vi "Controller test.vi"() -> ()   [LabVIEW 2018]
doc: "Test-bench for the various controllers and discrete transfer functions."
uses:
  TypeDefs/Select_TF.ctl
  <vilib>/Platform/TimedLoop/XDataNode/timing_clust.ctl
  <vilib>/Platform/TimedLoop/XDataNode/nitl_modes.ctl
  <vilib>/Platform/TimedLoop/XDataNode/wakeup.ctl
  Controllers/TF_diff_mode.ctl
  <vilib>/platform/TimedLoop/XDataNode/XDataNode.xnode
  <vilib>/Platform/TimedLoop/XDataNode/XDNodeRunTimeDep.lvlib
  Controllers/DiscreteControllers.lvlib
  <vilib>/ptbypt/NI_PtbyPt.lvlib
panel:
  in  "Select discrete \ntransfer function":T1
  out "#Loops late":i16
  in  "stop":bool
  out "System Waveform Chart":cluster{"square wave":dbl, "Output":dbl}(graph)
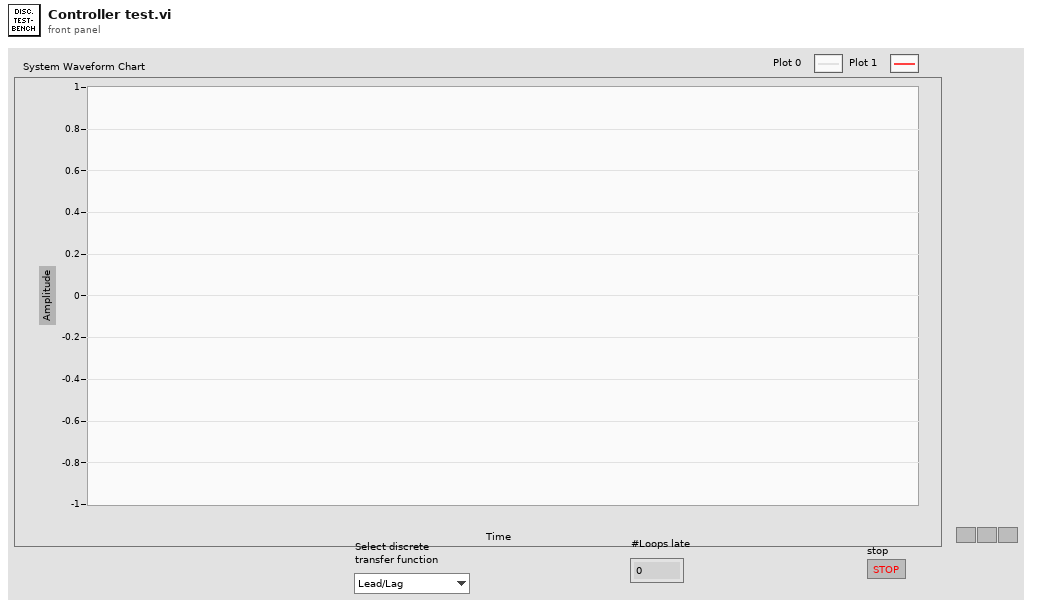
[diagram p1: front panel]
types:
  T1 = typedef "Select_TF.ctl" = enum16{"Lead/Lag", "Gain=20", "Unity", "Integrator"}
  T2 = typedef "XDNodeRunTimeDep.lvlib/timing_clust.ctl" = cluster{"Expected End [f-1]":u64, "Actual End [f-1]":u64, "Finished Late? [f-1]":bool, "Expected End [i-1]":u64, "Actual End [i-1]":u64, "Finished Late? [i-1]":bool, "Expected Start [i]":u64, "Actual Start [i]":u64, "Expected Start [f]":u64, "Actual Start [f]":u64, "Source Name":string, "Structure Name":string, "Period":i64, "Deadline":i64, "Offset":i64, "Start":i64, "Priority":i32, "Timeout":i32, "Mode":T3, "Wakeup Reason":T4, "Error":errorcluster, "Source Type":string, "Secondary Source Type":string, "Global End Time":u64, "Global Start Time":u64, "Frame Duration":u64, "Iteration Duration":u64, "Assigned CPU":i32, "I/O Scan Engine Mode":u32}
  T3 = typedef "XDNodeRunTimeDep.lvlib/nitl_modes.ctl" = enum32{"No Change", "Process missed periods, maintain original phase", "Discard missed periods, maintain original phase", "Process missed periods, ignore original phase", "Discard missed periods, ignore original phase"}
  T4 = typedef "XDNodeRunTimeDep.lvlib/wakeup.ctl" = enum32{"Normal", "Aborted", "Asynchronous wakeup", "Timing source error", "Timed loop error", "Timeout"}
  T5 = typedef "DiscreteControllers.lvlib/TF_diff_mode.ctl" = enum16{"Forward Euler", "Backward Euler", "Tustin (Bilinear)"}
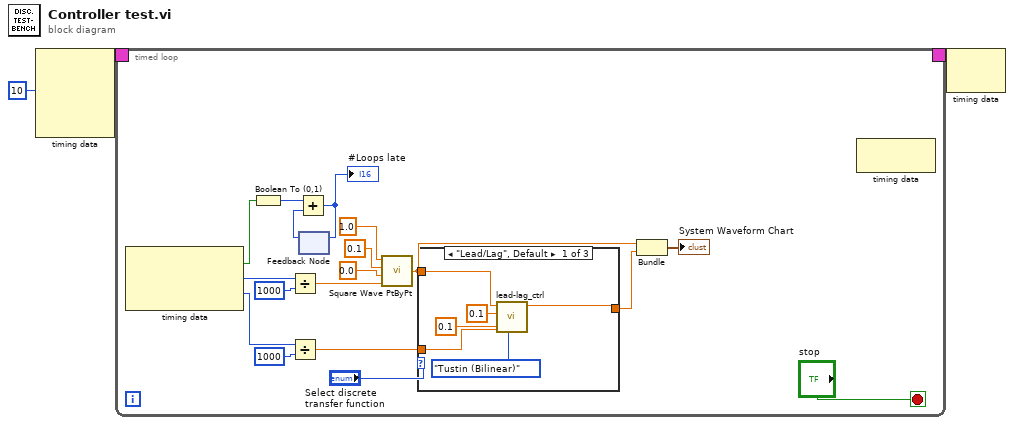
[diagram p0: block diagram]
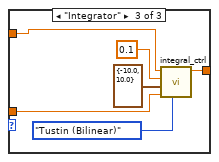
[diagram p3: hidden frame]
diagram:
  n1 = node-c288(i64 10 ("Period")) -> (w3:T2)  [unwired: 3 in]
  n2 = timed-loop {
    timing: w3 -> [_]
    timing-out: [_] -> w2
    stop <- "stop" stop-if-true
    n3 = node-c288() -> (w8:bool, w21:i64, w15:i64)  [unwired: 1 in]
    n4 = Boolean To (0,1)(Boolean=w8) -> (0, 1=w7:i16)
    n5 = Divide(x=w21, y=i64 1000) -> (x/y=w19:dbl)
    n6 = Divide(x=w15, y=i64 1000) -> (x/y=w13:dbl)
    n7 = feedback #1() -> (w5:i16)  [unwired: 1 in]
    n8 = Add(x=w7, y=w5) -> (x+y=w6:i16)
    "#Loops late" <- w6
    n9 = feedback-in #1(w6) -> ()
    n10 = call <vilib>:"Square Wave PtByPt.vi"("amplitude"=1.0, "frequency"=0.1, "phase"=0.0, "time"=w19) -> ("square wave"=w10:dbl)  [unwired: 1 in]
    n11 = case shown="\"Lead/Lag\", Default" "Select discrete \ntransfer function" {
      tunnel: w13 -> [w24 _ w32]
      tunnel: w10 -> [w27 w28 w30]
      tunnel: [w23 w28 w29] -> w9
      frame "Lead/Lag", Default {
        n12 = call "lead-lag_ctrl.vi"("Mode"=TF_diff_mode."Tustin (Bilinear)", "Sampling Time"=w24, "tau"=0.1, "alpha"=0.1, "Input"=w27) -> ("Output"=w23:dbl)  [unwired: 5 in, 1 out]
      }
      frame "Unity" {
      }
      frame "Integrator" {
        n13 = call "integral_ctrl.vi"("Mode"=TF_diff_mode."Tustin (Bilinear)", "Sampling \nTime"=w32, "Anti-windup limits"=cluster{"Lower limit":dbl, "Upper limit":dbl} {"Lower limit"=-10.0, "Upper limit"=10.0}, "Ki"=0.1, "Input"=w30) -> ("Output"=w29:dbl)  [unwired: 5 in, 1 out]
      }
    }
    n14 = Bundle("square wave"=w10, "Output"=w9) -> (→"System Waveform Chart":cluster{"square wave":dbl, "Output":dbl})  [unwired: 1 in]
    n15 = node-c288() -> ()  [unwired: 1 in, 1 out]
  }
  n16 = node-c288(w2) -> ()  [unwired: 1 out]
